vi "FilterOnMainPic.vi"(6 "Filters 4":T1(ring), 9 "right":i16, 10 "bottom":i16, 11 "Noised picture":picture) -> (3 "Noise+Pic 2":picture caption="filtered picture", 7 "Filtered X":dbl[](array[numeric]))   [LabVIEW 2016]
uses:
  <vilib>/Analysis/3filter.llb/Equi-Ripple LowPass (DBL).vi
  <vilib>/Analysis/3filter.llb/Equi-Ripple HighPass (DBL).vi
  <vilib>/Analysis/3filter.llb/Equi-Ripple BandPass (DBL).vi
  <vilib>/Analysis/3filter.llb/Equi-Ripple BandStop (DBL).vi
  <vilib>/Analysis/3filter.llb/Butterworth Filter (DBL).vi
  <vilib>/Analysis/NI_AALBase.lvlib
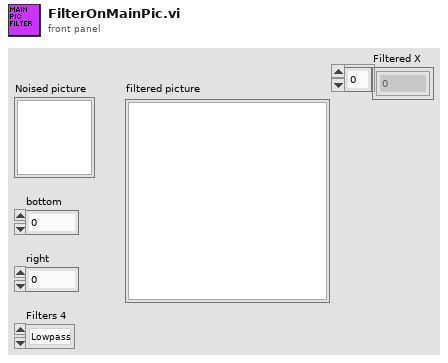
[diagram p1: front panel]
types:
  T1 = enum32{"Lowpass ", "Highpass", "Band pass", "Band Stop", "Butter Worth ", "No filter"}
  T2 = typedef "imagedata.ctl" = cluster{"image type":i32, "image depth":i32, "image":u8[], "mask":u8[], "colors":u32[], "Rectangle":cluster{"left":i16, "top":i16, "right":i16, "bottom":i16}}
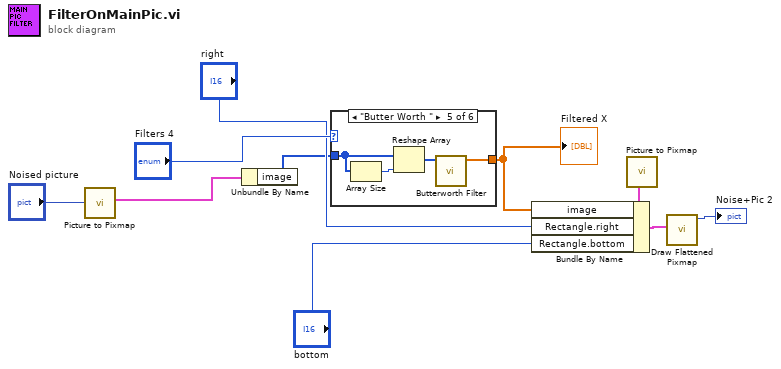
[diagram p0: block diagram]
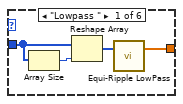
[diagram p2: hidden frame]
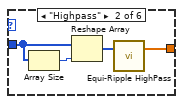
[diagram p3: hidden frame]
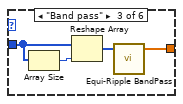
[diagram p4: hidden frame]
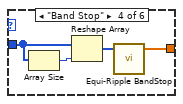
[diagram p5: hidden frame]
diagram:
  n1 = call <vilib>:"Picture to Pixmap.vi"("picture"="Noised picture") -> ("image data"=w2:T2)  [unwired: 9 in, 1 out]
  n2 = Unbundle By Name(w2) -> ("image"=w3:u8[])
  n3 = case shown="\"Butter Worth \"" "Filters 4" {
    tunnel: w3 -> [w12 w16 w20 w23 w29 w31]
    tunnel: [w11 w15 w19 w25 w27 w31] -> w4
    frame "Lowpass " {
      n4 = Array Size(array=w12) -> (size(s)=w14:i32)
      n5 = Reshape Array(w12, w14) -> (w13:u8[])
      n6 = call-poly <vilib>:"Equi-Ripple LowPass.vi"("X"=w13) -> ("Filtered X"=w11:dbl[])  [unwired: 5 in, 1 out]
    }
    frame "Highpass" {
      n7 = Array Size(array=w16) -> (size(s)=w18:i32)
      n8 = Reshape Array(w16, w18) -> (w17:u8[])
      n9 = call-poly <vilib>:"Equi-Ripple HighPass.vi"("X"=w17) -> ("Filtered X"=w15:dbl[])  [unwired: 5 in, 1 out]
    }
    frame "Band pass" {
      n10 = Array Size(array=w20) -> (size(s)=w22:i32)
      n11 = Reshape Array(w20, w22) -> (w21:u8[])
      n12 = call-poly <vilib>:"Equi-Ripple BandPass.vi"("X"=w21) -> ("Filtered X"=w19:dbl[])  [unwired: 7 in, 1 out]
    }
    frame "Band Stop" {
      n13 = Array Size(array=w23) -> (size(s)=w26:i32)
      n14 = Reshape Array(w23, w26) -> (w24:u8[])
      n15 = call-poly <vilib>:"Equi-Ripple BandStop.vi"("X"=w24) -> ("Filtered X"=w25:dbl[])  [unwired: 7 in, 1 out]
    }
    frame "Butter Worth " {
      n16 = Array Size(array=w29) -> (size(s)=w30:i32)
      n17 = Reshape Array(w29, w30) -> (w28:u8[])
      n18 = call-poly <vilib>:"Butterworth Filter.vi"("X"=w28) -> ("Filtered X"=w27:dbl[])  [unwired: 7 in, 1 out]
    }
    frame "No filter", Default {
    }
  }
  "Filtered X" <- w4
  n19 = call <vilib>:"Picture to Pixmap.vi"() -> ("image data"=w7:T2)  [unwired: 10 in, 1 out]
  n20 = Bundle By Name(cluster=w7, "image"=w4, "Rectangle.right"="right", "Rectangle.bottom"="bottom") -> (w8:T2)
  n21 = call <vilib>:"Draw Flattened Pixmap.vi"("image data"=w8) -> ("new picture"=→"Noise+Pic 2":picture)  [unwired: 8 in]
